vi "_Set FP Origin.vi"(8 "Error In":errorcluster, 10 "Origin (0,0)":cluster{"Horizontal":i16, "Verticle":i16}, 11 "VI Ref":refnum<vi>) -> (0 "Error Out":errorcluster)   [LabVIEW 2011, in "LVH-Build-Tools.lvlib"]
doc: "Set the specified VIs front panel origin position."
uses:
  LVH-Build-Tools.lvlib
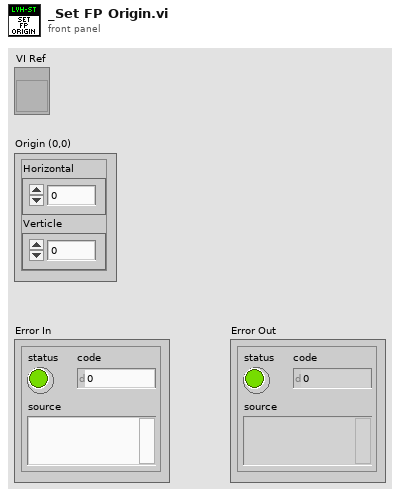
[diagram p1: front panel]
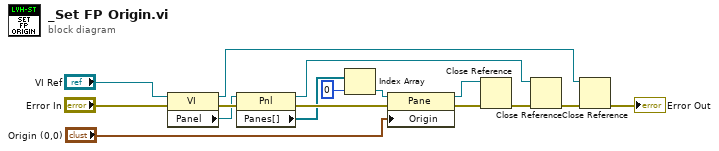
[diagram p0: block diagram]
diagram:
  n1 = property class="VI"(reference="VI Ref", error in="Error In") -> (reference out=w4:refnum<vi>, error out=w14:errorcluster, "Panel"=w9:refnum<vi>)
  n2 = property class="Pnl"(reference=w9, error in=w14) -> (reference out=w6:refnum<vi>, error out=w13:errorcluster, "Panes[]"=w10:refnum<vi>[])
  n3 = Index Array(array=w10, index=0) -> (element=w12:refnum<vi>)
  n4 = property class="Pane"(reference=w12, error in=w13, "Origin"="Origin (0,0)") -> (reference out=w7:refnum<vi>, error out=w8:errorcluster)
  n5 = Close Reference(reference=w7, error in (no error)=w8) -> (error out=w1:errorcluster)
  n6 = Close Reference(reference=w6, error in (no error)=w1) -> (error out=w5:errorcluster)
  n7 = Close Reference(reference=w4, error in (no error)=w5) -> (error out=→"Error Out":errorcluster)
